vi "Set_motor_direction.vi"(0 "TCP Network Connection in":refnum<k5>, 1 "Step status":bool, 5 "Step Count":i32, 7 "ADC distance":dbl, 9 "Cup Position":T2(ring), 11 "error in (no error)":errorcluster) -> (4 "TCP Network Connection out":refnum<k5>, 15 "error out":errorcluster)   [LabVIEW 2019]
panel:
  in  "Possition selector":T1(radio)
  out "element":dbl
  in  "ADC possitions":dbl[](array[numeric])=[6.31684, 27.7371, 181.99, 240.785, 293.499]
  in  "Step possitions":dbl[](array[numeric])=[-1280.0, -5428.0, -35785.0, -47327.0, -57601.0]
  out "Driver response":bool
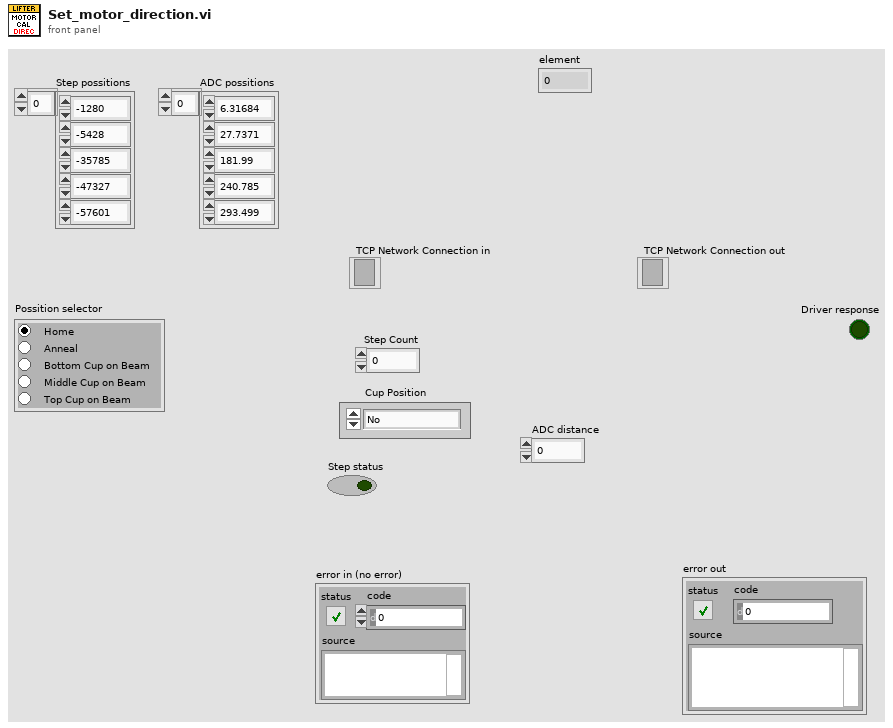
[diagram p1: front panel]
types:
  T1 = enum32{"Home", "Anneal", "Bottom Cup on Beam", "Middle Cup on Beam", "Top Cup on Beam"}
  T2 = enum16{"No", "Home", "Anneal", "Bottom Cup", "Middle Cup", "Top Cup"}
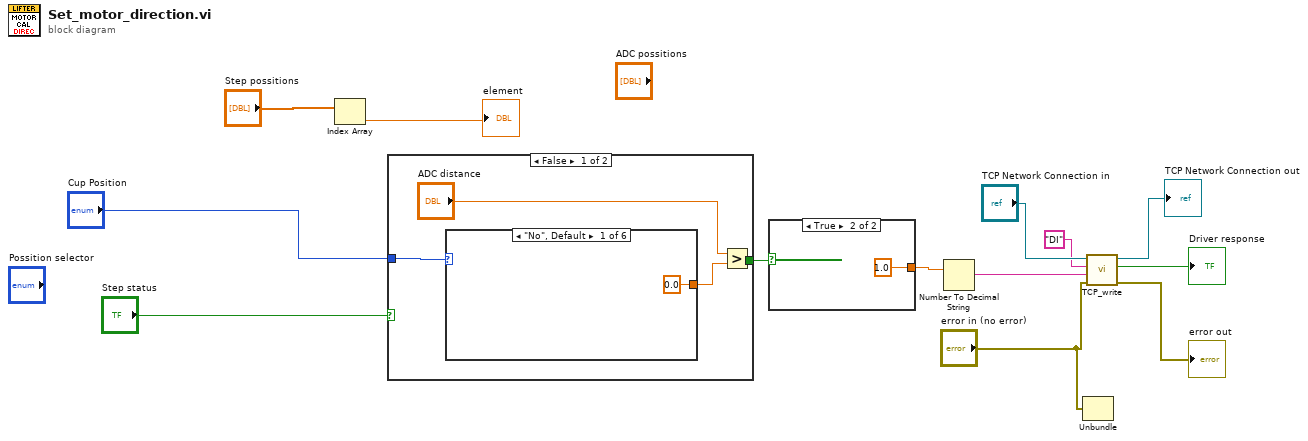
[diagram p0: block diagram]
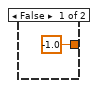
[diagram p2: hidden frame]
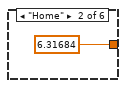
[diagram p3: hidden frame]
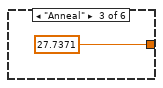
[diagram p4: hidden frame]
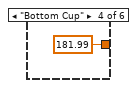
[diagram p5: hidden frame]
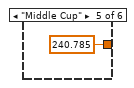
[diagram p6: hidden frame]
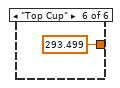
[diagram p7: hidden frame]
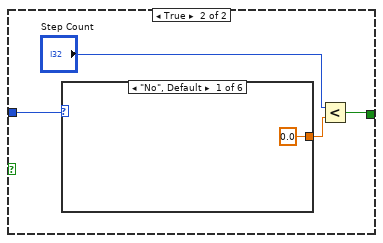
[diagram p8: hidden frame]
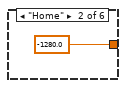
[diagram p9: hidden frame]
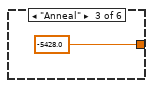
[diagram p10: hidden frame]
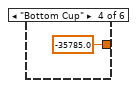
[diagram p11: hidden frame]
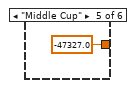
[diagram p12: hidden frame]
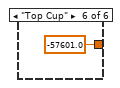
[diagram p13: hidden frame]
diagram:
  n1 = Index Array(array="Step possitions") -> (element=→"element":dbl)  [unwired: 1 in]
  n2 = case shown="False" "Step status" {
    tunnel: "Cup Position" -> [w17 w27]
    tunnel: [w14 w26] -> w11
    frame False {
      n3 = case shown="\"No\", Default" w17 {
        tunnel: [0.0 6.31684 27.7371 181.99 240.785 293.499] -> w16
        frame "No", Default {
        }
        frame "Home" {
        }
        frame "Anneal" {
        }
        frame "Bottom Cup" {
        }
        frame "Middle Cup" {
        }
        frame "Top Cup" {
        }
      }
      n4 = Greater?(x="ADC distance", y=w16) -> (0:w14:bool)
    }
    frame True {
      n5 = case shown="\"No\", Default" w27 {
        tunnel: [0.0 -1280.0 -5428.0 -35785.0 -47327.0 -57601.0] -> w25
        frame "No", Default {
        }
        frame "Home" {
        }
        frame "Anneal" {
        }
        frame "Bottom Cup" {
        }
        frame "Middle Cup" {
        }
        frame "Top Cup" {
        }
      }
      n6 = Less?(x="Step Count", y=w25) -> (x < y?=w26:bool)
    }
  }
  n7 = case shown="True" w11 {
    tunnel: [-1.0 ("Direction") 1.0 ("Direction")] -> w10
    frame False {
    }
    frame True {
    }
  }
  n8 = Number To Decimal String(number=w10) -> (decimal integer string=w7:string)  [unwired: 1 in]
  n9 = Unbundle("error in (no error)") -> ()  [unwired: 3 out]
  n10 = call "TCP_write.vi"("error in"="error in (no error)", "Parameter 2"=w7, "Parameter 1"="DI" ("string"), "connection ID"="TCP Network Connection in") -> ("error out"=→"error out":errorcluster, "Driver response"=→"Driver response":bool, "TCP Network Connection out"=→"TCP Network Connection out":refnum<k5>)  [unwired: 5 in]
